vi "Set Transceiver Loader.vi"(10 "Transceiver Loader":refnum<class "Transceiver Loader.lvclass">, 11 "Framework in":refnum<class "Framework.lvclass">) -> (3 "Framework out":refnum<class "Framework.lvclass">)   [LabVIEW 2017, in "Data Sharing Framework Core.lvlib" / "Data Sharing Framework Engine.lvlib" / "Framework.lvclass"]
uses:
  Framework.lvclass
  Internal/Transceiver/Transceiver Loader/Transceiver Loader.lvclass
  Framework.lvclass/Framework.ctl
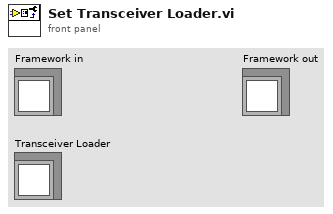
[diagram p1: front panel]
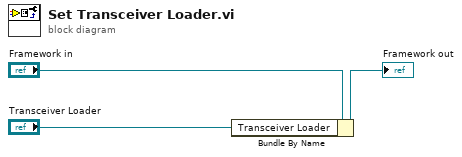
[diagram p0: block diagram]
diagram:
  n1 = Bundle By Name(cluster="Framework in", "Transceiver Loader"="Transceiver Loader") -> (→"Framework out":refnum<class "Framework.lvclass">)
